vi "Reply to Message.vi"(8 "error in (no error)":errorcluster, 10 "Message":string, 11 "0MQ_Server in":refnum<class "0MQ_Server.lvclass">) -> (0 "error out":errorcluster, 3 "0MQ_Server out":refnum<class "0MQ_Server.lvclass">)   [LabVIEW 2016, in "0MQ_Server.lvclass"]
uses:
  0MQ_Server.lvclass
  0MQ_Server.lvclass/0MQ_Server.ctl
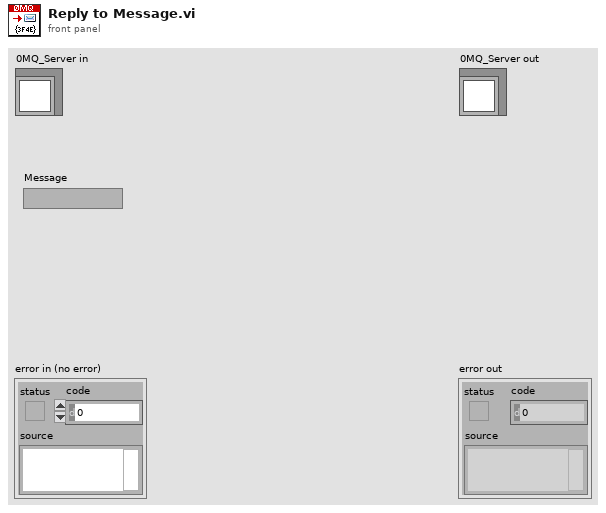
[diagram p1: front panel]
types:
  T1 = typedef "zeromq.lvlib/socket_type.ctl" = enum8{"ZMQ_PAIR", "ZMQ_PUB", "ZMQ_SUB", "ZMQ_REQ", "ZMQ_REP", "ZMQ_DEALER", "ZMQ_ROUTER", "ZMQ_PULL", "ZMQ_PUSH", "ZMQ_XPUB", "ZMQ_XSUB"}
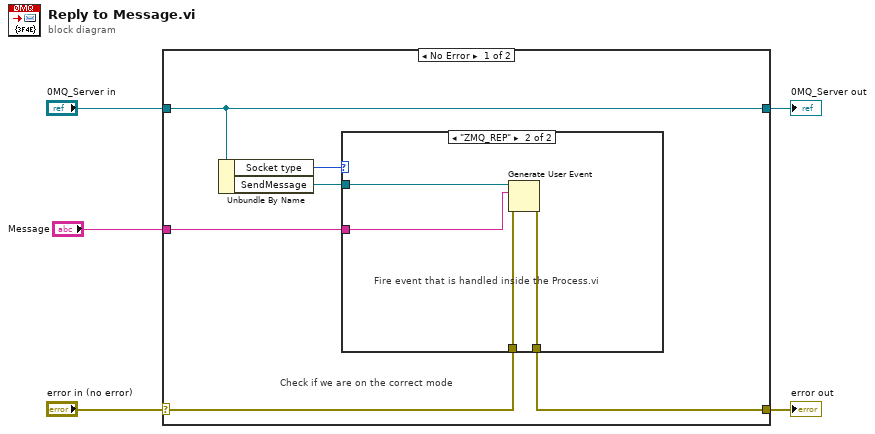
[diagram p0: block diagram]
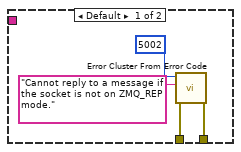
[diagram p2: hidden frame]
diagram:
  n1 = case shown="No Error" "error in (no error)" {
    selector: "error in (no error)" -> [w10 w21]
    tunnel: [w9 w21] -> w4
    tunnel: [w11 w20] -> w2
    tunnel: "0MQ_Server in" -> [w11 w20]
    tunnel: "Message" -> [w7 _]
    frame No Error {
      # "Check if we are on the correct mode"
      n2 = Unbundle By Name(w11) -> ("Socket type"=w6:T1, "SendMessage"=w8:refnum<user-event>)
      n3 = case shown="\"ZMQ_REP\"" w6 {
        tunnel: w10 -> [w15 w19]
        tunnel: [w14 w18] -> w9
        tunnel: w8 -> [_ w17]
        tunnel: w7 -> [_ w16]
        frame Default {
          n4 = call <vilib>:"Error Cluster From Error Code.vi"("error in (no error)"=w15, "error message (\"\")"="Cannot reply to a message if the socket is not on ZMQ_REP mode." ("error message (\"\")"), "error code (0)"=5002) -> ("error out"=w14:errorcluster)  [unwired: 6 in]
        }
        frame "ZMQ_REP" {
          # "Fire event that is handled inside the Process.vi"
          n5 = Generate User Event(user event=w17, event data cluster=w16, error in=w19) -> (error out=w18:errorcluster)  [unwired: 1 in, 1 out]
        }
      }
    }
    frame Error {
    }
  }
  "error out" <- w4
  "0MQ_Server out" <- w2
